vi "Allow Access to onenote.vi"(8 "error in (no error)":errorcluster) -> (0 "error out":errorcluster, 3 "LocationURL":string)   [LabVIEW 2016]
panel:
  in  "WebBrowser":refnum<k7>(container)
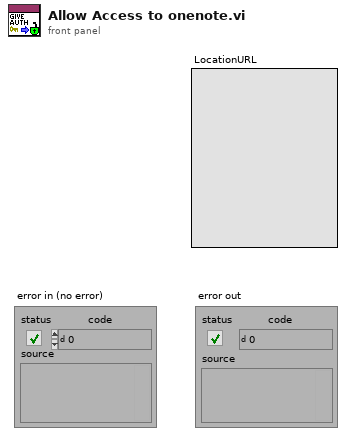
[diagram p1: front panel]
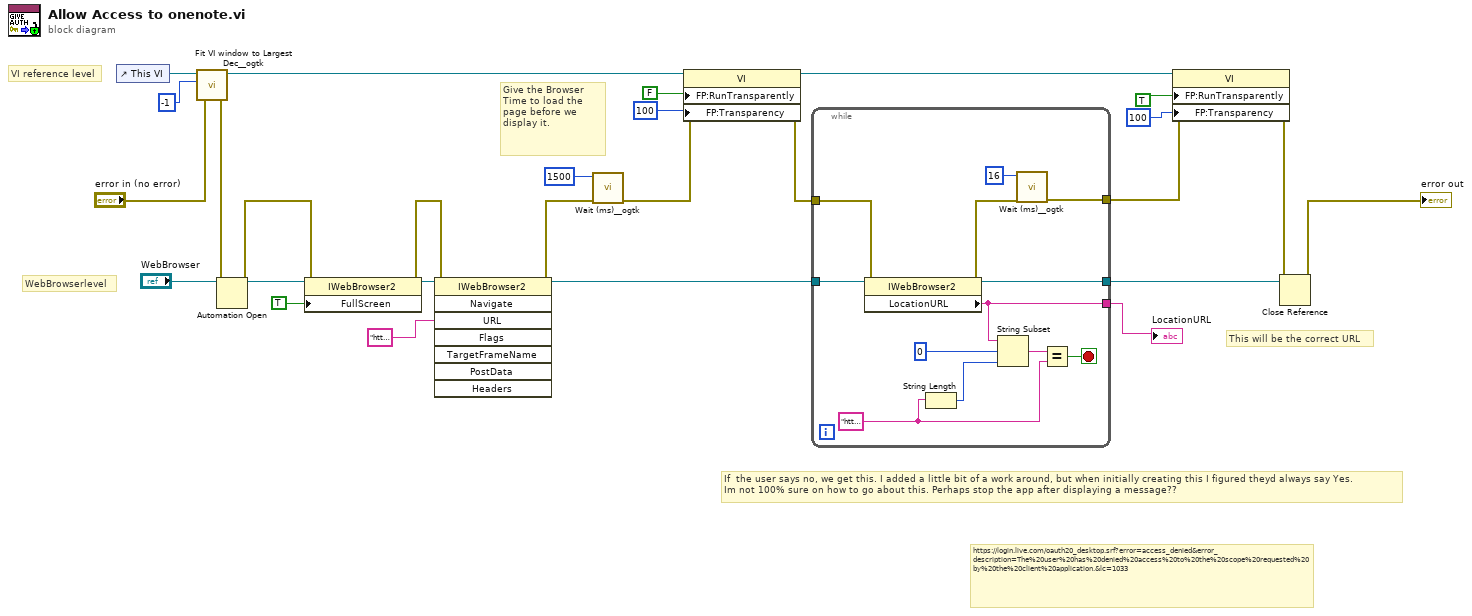
[diagram p0: block diagram]
diagram:
  # "VI reference level"
  # "WebBrowserlevel"
  # "If  the user says no, we get this. I added a little bit of a work around, but when initially creating this I figured theyd always say Yes.\nIm not 100% sure on how to go about this. Perhaps stop the app after displaying a message??"
  # "https://login.live.com/oauth20_desktop.srf?error=access_denied&error_description=The%20user%20has%20denied%20access%20to%20the%20scope%20requested%20by%20the%20client%20application.&lc=1033"
  # "Give the Browser Time to load the page before we display it."
  # "This will be the correct URL"
  n1 = control-ref of="This VI"() -> (w15:refnum<vi>)
  n2 = call <userlib>:"Fit VI window to Largest Dec__ogtk.vi"("error in (no error)"="error in (no error)", "border spacing (2 px)"=-1, "VI Ref (calling VI)"=w15) -> ("error out"=w12:errorcluster, "dup VI Ref"=w14:refnum<vi>)  [unwired: 3 in]
  n3 = Automation Open(error in (no error)=w12, Automation Refnum="WebBrowser") -> (Automation Refnum=w27:refnum<k7>, error out=w11:errorcluster)  [unwired: 2 in]
  n4 = property class="IWebBrowser2"(reference=w27, error in=w11, "FullScreen"=TRUE) -> (reference out=w25:refnum<k7>, error out=w10:errorcluster)
  n5 = invoke class="IWebBrowser2" method="Navigate"(reference=w25, error in=w10, "URL"="https://login.live.com/oauth20_authorize.srf?response_type=code&client_id=c698ce01-75b1-4eb8-b040-9787b75e6b48&redirect_uri=https://login.live.com/oauth20_desktop.srf&scope=office.onenote_update&scope=wl.offline_access") -> (reference out=w5:refnum<k7>, error out=w9:errorcluster)  [unwired: 5 in, 6 out]
  n6 = call <userlib>:"Wait (ms)__ogtk.vi"("error in (no error)"=w9, "milliseconds to wait"=u32 1500) -> ("error out"=w8:errorcluster)  [unwired: 8 in, 1 out]
  n7 = property class="VI"(reference=w14, error in=w8, "FP:RunTransparently"=FALSE ("Front Panel Window:Run VI Transparently"), "FP:Transparency"=u8 100 ("Front Panel Window:Transparency")) -> (reference out=w7:refnum<vi>, error out=w4:errorcluster)
  n8 = while {
    tunnel: [w39] -> w6
    tunnel: [w32] -> w21
    tunnel: w5 -> [w31]
    tunnel: w4 -> [w30]
    tunnel: [w28] -> w1
    stop <- w35 stop-if-true
    w33 = "https://login.live.com/oauth20_desktop.srf"
    n9 = property class="IWebBrowser2"(reference=w31, error in=w30) -> (reference out=w39:refnum<k7>, error out=w29:errorcluster, "LocationURL"=w32:string)
    n10 = String Length(string=w33) -> (length=w38:i32)
    n11 = String Subset(string=w32, offset (0)=0, length (rest)=w38) -> (substring=w36:string)
    n12 = call <userlib>:"Wait (ms)__ogtk.vi"("error in (no error)"=w29, "milliseconds to wait"=u32 16) -> ("error out"=w28:errorcluster)  [unwired: 8 in, 1 out]
    n13 = Equal?(x=w36, y=w33) -> (x = y?=w35:bool)
  }
  "LocationURL" <- w21
  n14 = property class="VI"(reference=w7, error in=w1, "FP:RunTransparently"=TRUE ("Front Panel Window:Run VI Transparently"), "FP:Transparency"=u8 100 ("Front Panel Window:Transparency")) -> (error out=w2:errorcluster)  [unwired: 1 out]
  n15 = Close Reference(reference=w6, error in (no error)=w2) -> (error out=→"error out":errorcluster)
